vi "Conjugate Quaternion.vi"(1 "quaternion":T1) -> (0 "conjugate":T1)   [LabVIEW 2017, in "NI_Kinematics.lvlib"]
doc: "Returns the conjugate of a quaternion."
uses:
  <vilib>/robotics/Kinematics/NI_Kinematics.lvlib
  <vilib>/robotics/Kinematics/Quaternion.ctl
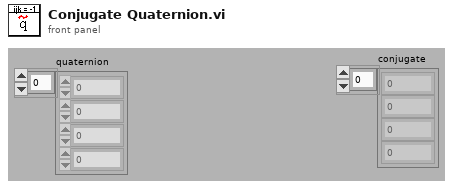
[diagram p1: front panel]
types:
  T1 = typedef "NI_Kinematics.lvlib/Quaternion.ctl" = dbl[]
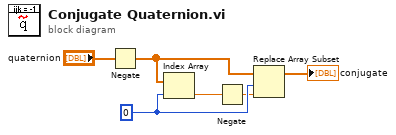
[diagram p0: block diagram]
diagram:
  w6 = 0 ("index")
  n1 = Negate(x="quaternion") -> (-x=w2:T1)
  n2 = Index Array(array=w2, index=w6) -> (element=w4:dbl)
  n3 = Negate(x=w4) -> (-x=w5:dbl)
  n4 = Replace Array Subset(array=w2, new element=w5, index=w6) -> (→"conjugate":T1)
